vi "Read Instrument ID.vi"(8 "error in (no error)":errorcluster, 11 "Instrument Owner in":refnum<class "Instrument Owner.lvclass">) -> (0 "error out":errorcluster, 2 "Instrument ID out":u32, 3 "Instrument Owner out":refnum<class "Instrument Owner.lvclass">)   [LabVIEW 2020, in "Instrument Handler.lvlib" / "Instrument Owner.lvclass"]
doc: "This VI exposes the Instrument Read to the Community Scope."
uses:
  Instrument Owner.lvclass
  Instrument Owner.lvclass/Instrument Owner.ctl
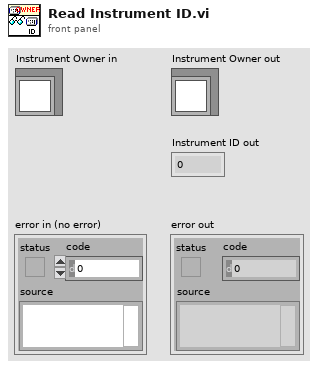
[diagram p1: front panel]
types:
  T1 = typedef "Instrument Handler.lvlib/Ctl_InstrumentSynchronicationCluster.ctl" = cluster{"Launched?":bool, "Driver Path":path, "Alias":string, "Connection Type":T2, "Pre Initialization Data":variant, "Enqueue Sync":refnum<class "Notifier.lvclass">, "Enqueue Lock":T3, "Owner Enqueuer":refnum<class "Message Enqueuer.lvclass">, "Owner":refnum<class "Sequencer Core.lvclass">, "Instrument ID":u32}
  T2 = typedef "HDH.Actor Framework.Core.Instrument Driver.lvlibp/Instrument Driver.lvclass/Ctl_ConnectionType.ctl" = enum16{"BuiltIn/System", "PXI/PCI", "USB", "GPIB", "VXI", "Serial", "TCP/IP", "cRIO", "SCXI", "cDAQ", "SwitchBlock", "SCC", "FireWire", "Accessory", "CAN", "SwitchBlock Device"}
  T3 = typedef "Semaphore RefNum" = refnum<k1>
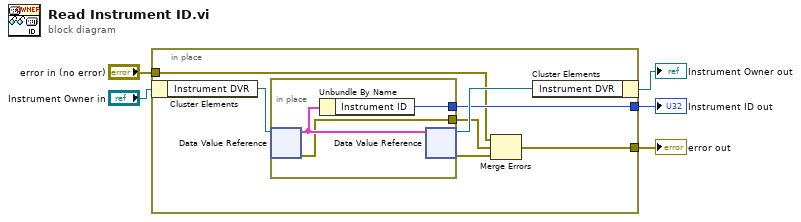
[diagram p0: block diagram]
diagram:
  n1 = in-place {
    in-place-border: [w10] -> w4
    in-place-border: "error in (no error)" -> [w7]
    in-place-border: [w6] -> w2
    n2 = in-place-cluster #1("Instrument Owner in") -> ("Instrument DVR"=w12:refnum<data-value>)
    n3 = in-place {
      in-place-border: [w14] -> w10
      in-place-border: [w13] -> w9
      n4 = in-place-dvr #2(w12) -> (w15:T1, w13:errorcluster)
      n5 = Unbundle By Name(w15) -> ("Instrument ID"=w14:u32)
      n6 = in-place-dvr #2(w15) -> (w11:refnum<data-value>, w8:errorcluster)
    }
    n7 = Merge Errors(w7, w9, w8) -> (w6:errorcluster)
    n8 = in-place-cluster #1("Instrument DVR"=w11) -> (→"Instrument Owner out":refnum<class "Instrument Owner.lvclass">)
  }
  "error out" <- w2
  "Instrument ID out" <- w4
